vi "belt control.vi"(1 "State":T1, 2 "Joystick Z":dbl) -> (0 "output":dbl)   [LabVIEW 2013]
uses:
  typedefs/subStates.ctl
  typedefs/fg_typedef.ctl
panel:
  in  "Time to Wait":u32
  in  "Rate":dbl=0.8 format="%#_13g"
  in  "upper limit":dbl=0.015 format="%#_13g"
  in  "lower limit":dbl=-0.015 format="%#_13g"
  # "Things to Tune"
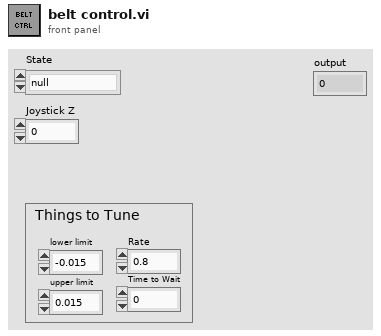
[diagram p1: front panel]
types:
  T1 = typedef "subStates.ctl" = enum16{"null", "wait", "driver control", "auto", "manual override", "hold position", "rotate", "pickup", "pass", "load", "goto shoot", "shoot", "cancel", "end"}
  T2 = typedef "fg_typedef.ctl" = enum16{"Get", "Set"}
  T3 = typedef "WPI_DigitalInputDevRef.ctl" = cluster{"DevStatus":errorcluster, "DIO Channel":T4, "Digital Module":T5}
  T4 = typedef "FPGA_DIOChannel.ctl" = enum8{"DIO 1", "DIO 2", "DIO 3", "DIO 4", "DIO 5", "DIO 6", "DIO 7", "DIO 8", "DIO 9", "DIO 10", "DIO 11", "DIO 12", "DIO 13", "DIO 14", "Invalid"}
  T5 = typedef "FPGA_TypedefDigitalModule.ctl" = enum16{"Digital Module 1", "Digital Module 2"}
  T6 = typedef "WPI_EncoderDevRef.ctl" = cluster{"DevStatus":errorcluster, "EncoderIndex":T7, "CounterIndex":T8, "DistancePerCount":dbl, "Decoding Type":T9}
  T7 = typedef "FPGA_EncoderIdx.ctl" = enum8{"Enc 0", "Enc 1", "Enc 2", "Enc 3", "Invalid"}
  T8 = typedef "FPGA_CounterCtrSystemIndex.ctl" = enum8{"Ctr 0", "Ctr 1", "Ctr 2", "Ctr 3", "Ctr 4", "Ctr 5", "Ctr 6", "Ctr 7", "Invalid"}
  T9 = typedef "WPI_EncoderType.ctl" = enum16{"1x", "2x", "4x"}
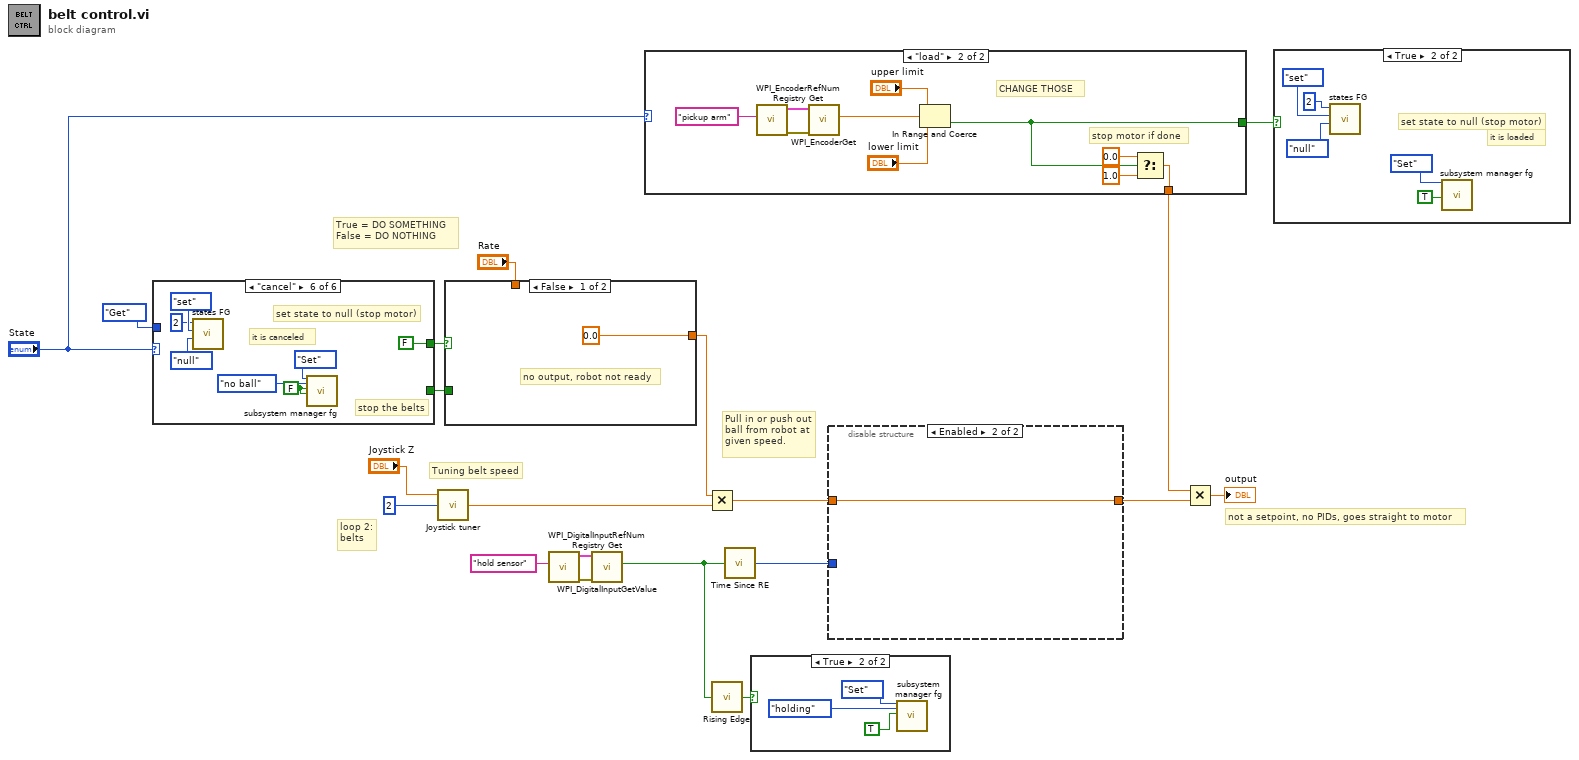
[diagram p0: block diagram]
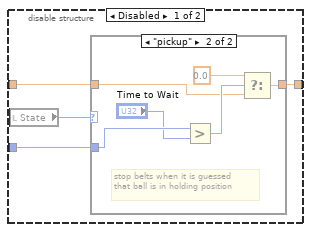
[diagram p2: hidden frame]
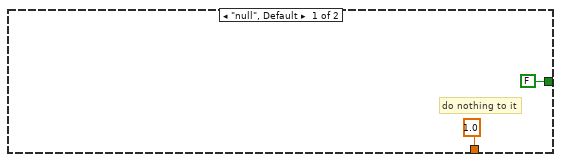
[diagram p5: hidden frame]
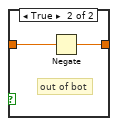
[diagram p8: hidden frame]
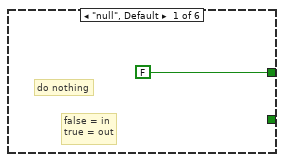
[diagram p9: hidden frame]
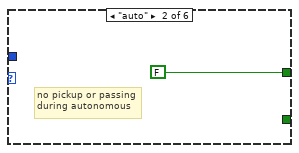
[diagram p10: hidden frame]
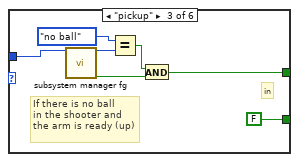
[diagram p11: hidden frame]
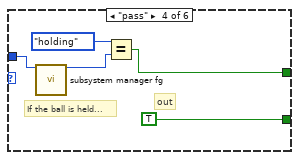
[diagram p12: hidden frame]
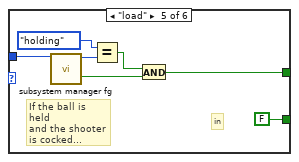
[diagram p13: hidden frame]
diagram:
  # "Pull in or push out\nball from robot at\ngiven speed."
  # "True = DO SOMETHING\nFalse = DO NOTHING"
  # "not a setpoint, no PIDs, goes straight to motor"
  # "Tuning belt speed"
  # "loop 2:\nbelts"
  n1 = case shown="\"cancel\"" "State" {
    tunnel: fg_typedef."Get" ("Menu") -> [_ _ w29 w34 w41 _]
    tunnel: [FALSE ("Arm Ready") FALSE ("Arm Ready") w23 w31 w36 FALSE ("Arm Ready")] -> w19
    tunnel: [_ _ FALSE TRUE FALSE _] -> w17
    frame "null", Default {
      # "false = in\ntrue = out"
      # "do nothing"
    }
    frame "auto" {
      # "no pickup or passing\nduring autonomous"
    }
    frame "pickup" {
      # "in"
      # "If there is no ball\nin the shooter and\nthe arm is ready (up)"
      n2 = call "subsystem manager fg.vi"("Menu"=w29) -> ("Ball State Read"=w26:enum16{"no ball", "holding", "loaded"}, "Arm Ready"=w24:bool)  [unwired: 14 in, 3 out]
      n3 = Equal?(x=enum16{"no ball", "holding", "loaded"}."no ball" ("y"), y=w26) -> (x = y?=w25:bool)
      n4 = And(x=w25, y=w24) -> (x .and. y?=w23:bool)
    }
    frame "pass" {
      # "out"
      # "If the ball is held..."
      n5 = call "subsystem manager fg.vi"("Menu"=w34) -> ("Ball State Read"=w32:enum16{"no ball", "holding", "loaded"})  [unwired: 14 in, 4 out]
      n6 = Equal?(x=enum16{"no ball", "holding", "loaded"}."holding" ("Ball State Read"), y=w32) -> (x = y?=w31:bool)
    }
    frame "load" {
      # "in"
      # "If the ball is held\nand the shooter\nis cocked..."
      n7 = call "subsystem manager fg.vi"("Menu"=w41) -> ("Ball State Read"=w39:enum16{"no ball", "holding", "loaded"}, "Shooter Cocked"=w35:bool)  [unwired: 14 in, 3 out]
      n8 = Equal?(x=enum16{"no ball", "holding", "loaded"}."holding" ("y"), y=w39) -> (x = y?=w37:bool)
      n9 = And(x=w37, y=w35) -> (x .and. y?=w36:bool)
    }
    frame "cancel" {
      w42 = FALSE ("Picked Up")
      # "it is canceled"
      # "set state to null (stop motor)"
      # "stop the belts"
      n10 = call "states FG.vi"("subState in"=subStates."null", "menu (get)"=enum16{"set", "get"}."set", "Loop ID"=2) -> ()  [unwired: 5 in, 4 out]
      n11 = call "subsystem manager fg.vi"("Menu"=fg_typedef."Set", "Ball State Write"=enum16{"no ball", "holding", "loaded"}."no ball", "Picked Up"=w42, "Loaded"=w42) -> ()  [unwired: 11 in, 5 out]
    }
  }
  n12 = call "Joystick tuner.vi"("Joystick Z"="Joystick Z", "Loop ID"=2) -> ("Output"=w1:dbl)  [unwired: 7 in]
  n13 = case shown="False" w19 {
    tunnel: [0.0 ("f") w51] -> w18
    tunnel: w17 -> [_ w52]
    tunnel: "Rate" -> [_ w50]
    frame False {
      # "no output, robot not ready"
    }
    frame True {
      n14 = case shown="False" w52 {
        tunnel: [w53 w55] -> w51
        tunnel: w50 -> [w53 w54]
        frame False {
          # "into bot"
        }
        frame True {
          # "out of bot"
          n15 = Negate(x=w54) -> (-x=w55:dbl)
        }
      }
    }
  }
  n16 = call <vilib>:"WPI_DigitalInputRefNum Registry Get.vi"("refnum name"="hold sensor") -> ("error out"=w16:errorcluster, "DigitalInputDevRef"=w15:T3)  [unwired: 9 in]
  n17 = call <vilib>:"WPI_DigitalInputGetValue.vi"("error in (no error)"=w16, "DigitalInputDevRef"=w15) -> ("Value"=w9:bool)  [unwired: 7 in, 2 out]
  n18 = case shown="\"load\"" "State" {
    tunnel: [FALSE w60] -> w12
    tunnel: [1.0 w61] -> w10
    frame "null", Default {
      # "do nothing to it"
    }
    frame "load" {
      # "stop motor if done"
      # "CHANGE THOSE"
      n19 = call <vilib>:"WPI_EncoderRefNum Registry Get.vi"("refnum name"="pickup arm") -> ("error out"=w65:errorcluster, "EncoderDevRef"=w66:T6)  [unwired: 9 in]
      n20 = call <vilib>:"WPI_EncoderGet.vi"("error in (no error)"=w65, "EncoderDevRef"=w66) -> ("Distance"=w62:dbl)  [unwired: 4 in, 5 out]
      n21 = In Range and Coerce(upper limit="upper limit", x=w62, lower limit="lower limit") -> (In Range?=w60:bool)  [unwired: 1 out]
      n22 = Select(t=0.0, s=w60, f=1.0) -> (s? t:f=w61:dbl)
    }
  }
  n23 = Multiply(x=w18, y=w1) -> (x*y=w6:dbl)
  n24 = call "Rising Edge.vi"("Input"=w9) -> ("Rising Edge"=w8:bool)
  n25 = call "Time Since RE.vi"("Input"=w9) -> ("Time Since RE of Input"=w4:u32)
  n26 = case shown="True" w8 {
    frame False {
    }
    frame True {
      n27 = call "subsystem manager fg.vi"("Menu"=fg_typedef."Set", "Ball State Write"=enum16{"no ball", "holding", "loaded"}."holding", "Picked Up"=TRUE) -> ()  [unwired: 12 in, 5 out]
    }
  }
  n28 = disable-structure shown="Enabled" {
    disable-tunnel: w6 -> [w73 w82]
    disable-tunnel: [w72 w82] -> w5
    disable-tunnel: w4 -> [w71 _]
    frame Disabled {
      n29 = local read "State"() -> (w74:T1)
      n30 = case shown="\"pickup\"" w74 {
        tunnel: w73 -> [w75 w77]
        tunnel: [w75 w79] -> w72
        tunnel: w71 -> [_ w81]
        frame "null", Default {
        }
        frame "pickup" {
          # "stop belts when it is guessed\nthat ball is in holding position"
          n31 = Greater?(x=w81, y="Time to Wait") -> (0:w78:bool)
          n32 = Select(t=0.0, s=w78, f=w77) -> (s? t:f=w79:dbl)
        }
      }
    }
    frame Enabled {
    }
  }
  n33 = Multiply(x=w10, y=w5) -> (x*y=→"output":dbl)
  n34 = case shown="True" w12 {
    frame False {
    }
    frame True {
      # "it is loaded"
      # "set state to null (stop motor)"
      n35 = call "states FG.vi"("subState in"=subStates."null", "menu (get)"=enum16{"set", "get"}."set", "Loop ID"=2) -> ()  [unwired: 5 in, 4 out]
      n36 = call "subsystem manager fg.vi"("Menu"=fg_typedef."Set", "Loaded"=TRUE) -> ()  [unwired: 13 in, 5 out]
    }
  }
